vi "RunOperation.vi"(10 "Inputs":string[](array[string]), 11 "BuildFromSource in":refnum<class "CiPipeline.lvclass">) -> (1 "Output/Failure":string, 2 "CLI Process Return Code":i32, 3 "BuildFromSource out":refnum<class "CiPipeline.lvclass">)   [LabVIEW 2024, in "CiPipeline.lvclass"]
uses:
  CiPipeline.lvclass
  CiPipeline.lvclass/CiPipeline.ctl
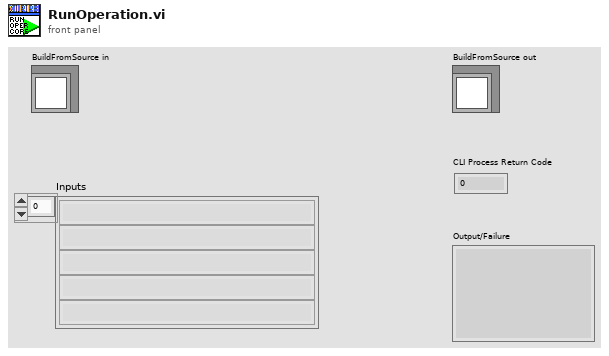
[diagram p1: front panel]
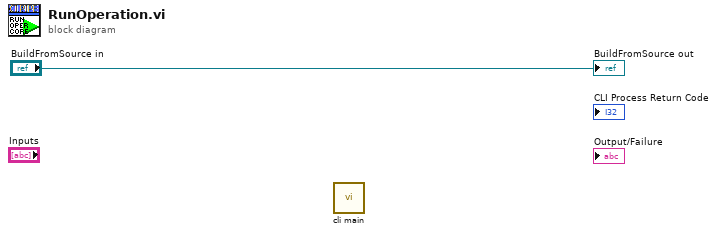
[diagram p0: block diagram]
diagram:
  n1 = call "cli main.vi"() -> ()  [unwired: 10 in, 2 out]
  "BuildFromSource out" <- "BuildFromSource in"
